vi "alinha-com-parede.vi"(4 "NXT/EV3":T2) -> (1 "NXT/EV3 2":T2)   [LabVIEW 2016]
uses:
  <vilib>/NXT/Subs/LVHSConnector.ctl
  <vilib>/NXT/LegoClasses/BrickReference/BrickReference.lvclass
  <vilib>/NXT/Block Support/NXT_InputPort.ctl
  <vilib>/NXT/Block Support/NXT_OutputPort.ctl
  <vilib>/NXT/Dual Mode Library/Sensors/Touch_Pressed.vi
  <vilib>/NXT/NXTIO Xnodes/NXTIONodeSubVIs/NXTMoveMotors.vi
  <vilib>/NXT/NXTIO Xnodes/AddressXNode/NXTIOAddress.xnode
  <vilib>/NXT/NXTIO Xnodes/NXTIOXNode/NXTIO.xnode
panel:
  in  "PortGyro":T1 items=["Port 1", "Port 2", "Port 3", "Port 4"]
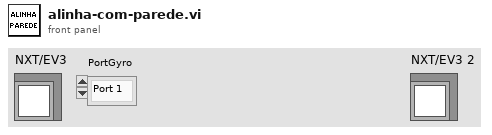
[diagram p1: front panel]
types:
  T1 = typedef "NXT_InputPort.ctl" = u32
  T2 = typedef "LVHSConnector.ctl" = refnum<class "BrickReference.lvclass">
  T3 = typedef "NXT_OutputPort.ctl" = u8
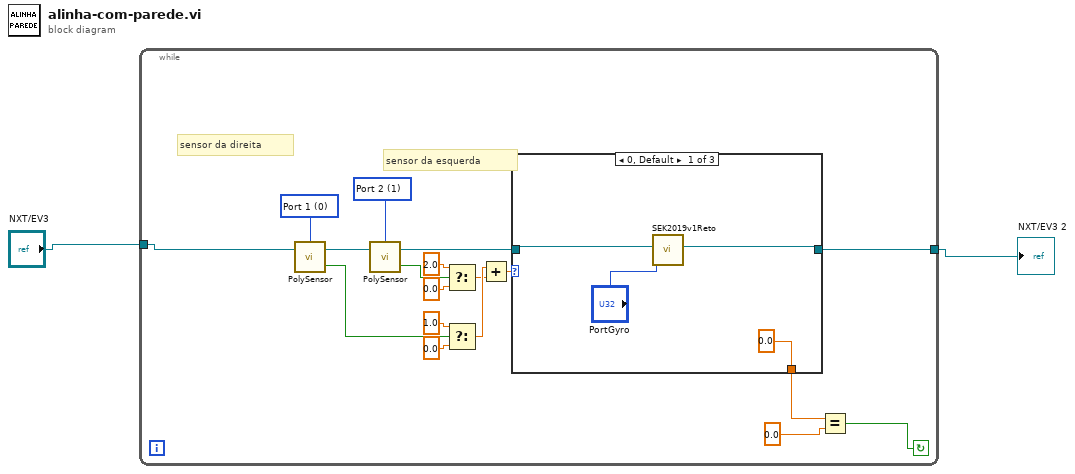
[diagram p0: block diagram]
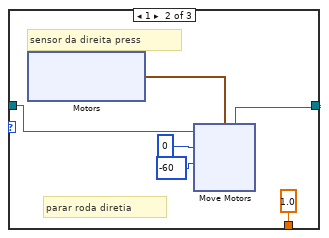
[diagram p2: hidden frame]
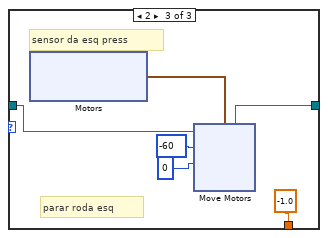
[diagram p3: hidden frame]
diagram:
  n1 = while {
    tunnel: "NXT/EV3" -> [w7]
    tunnel: [w6] -> w1
    stop <- w3 continue-if-true
    w19 = T1 1 items=["Port 1", "Port 2", "Port 3", "Port 4"] ("Port (Port 1)")
    w20 = T1 0 items=["Port 1", "Port 2", "Port 3", "Port 4"] ("Port (Port 1)")
    # "sensor da esquerda"
    # "sensor da direita"
    n2 = call-poly <vilib>:"PolySensor.vi"("NXT/EV3"=w7, "Port (Port 1)"=w20) -> ("Yes / No"=w17:bool, "NXT/EV3"=w18:T2)  [unwired: 1 in]
    n3 = call-poly <vilib>:"PolySensor.vi"("NXT/EV3"=w18, "Port (Port 1)"=w19) -> ("Yes / No"=w12:bool, "NXT/EV3"=w8:T2)  [unwired: 1 in]
    n4 = Select(t=2.0, s=w12, f=0.0 ("t")) -> (s? t:f=w10:dbl)
    n5 = Select(t=1.0, s=w17, f=0.0 ("t")) -> (s? t:f=w11:dbl)
    n6 = Add(x=w11, y=w10) -> (x+y=w9:dbl)
    n7 = case shown="0, Default" w9 {
      tunnel: w8 -> [w22 w27 w42]
      tunnel: [w23 w26 w41] -> w6
      tunnel: [0.0 ("t") 1.0 ("t") -1.0 ("t")] -> w5
      frame 0, Default {
        n8 = call "SEK2019v1Reto.vi"("NXT/EV3"=w22, "PortGyro"="PortGyro") -> ("NXT/EV3 2"=w23:T2)  [unwired: 9 in]
      }
      frame 1 {
        # "parar roda diretia"
        # "sensor da direita press"
        n9 = xnode "Motors"() -> ("Motor"=w28:cluster{"Port":T3, "Port":T3})
        n10 = xnode "Move Motors"("Power/Speed 2"=i8 -60, "Power/Speed 1"=i8 0, "Motors"=w28, "NXT/EV3"=w27) -> ("NXT/EV3"=w26:T2)
      }
      frame 2 {
        # "parar roda esq"
        # "sensor da esq press"
        n11 = xnode "Motors"() -> ("Motor"=w45:cluster{"Port":T3, "Port":T3})
        n12 = xnode "Move Motors"("Power/Speed 2"=i8 0 ("Power/Speed 1"), "Power/Speed 1"=i8 -60 ("Power/Speed 2"), "Motors"=w45, "NXT/EV3"=w42) -> ("NXT/EV3"=w41:T2)
      }
    }
    n13 = Equal?(x=w5, y=0.0 ("t")) -> (x = y?=w3:bool)
  }
  "NXT/EV3 2" <- w1
